vi "Mix Columns-PORTABLE-5129.vi"(7 "State In":u16[][](array[numeric])=[[45, 83, 174, 45], [73, 86, 101, 162], [176, 106, 51, 68], [108, 81, 250, 240]], 11 "error in":errorcluster) -> (8 "State Out":u16[][](array[numeric]), 15 "error out":errorcluster)   [LabVIEW 2020, in "Library Commun.lvlib"]
doc: "In the MixColumns step, the four bytes of each column of the state are combined using an invertible linear transformation. The MixColumns step can also be viewed as a multiplication by a particular MDS matrix in a finite field.\n\n<inline>"
uses:
  Library Commun.lvlib
panel:
  in  "0x011b":u16=283 format="%.0x"
  in  "0x80":u16=128 format="%.0x"
  # "old s= 45,83,174,45,73,86,101,162,176,106,51,68,108,81,250,240"
  # "new s= 93,103,33,19,24,16,203,78,171,34,184,12,86,107,80,106"
  # "255,97,23,96,160,73,200,160,172,154,205,24,        180,50,93,135"
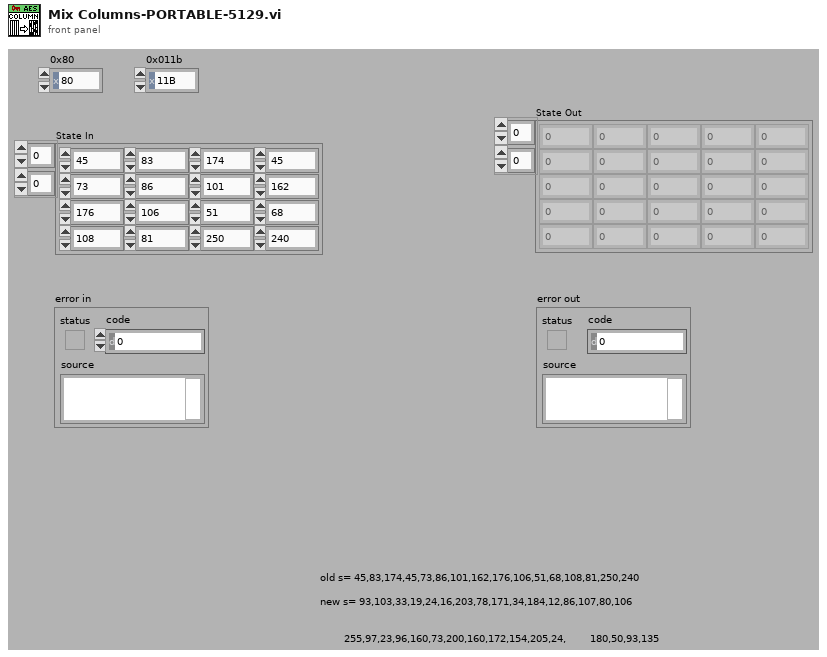
[diagram p1: front panel]
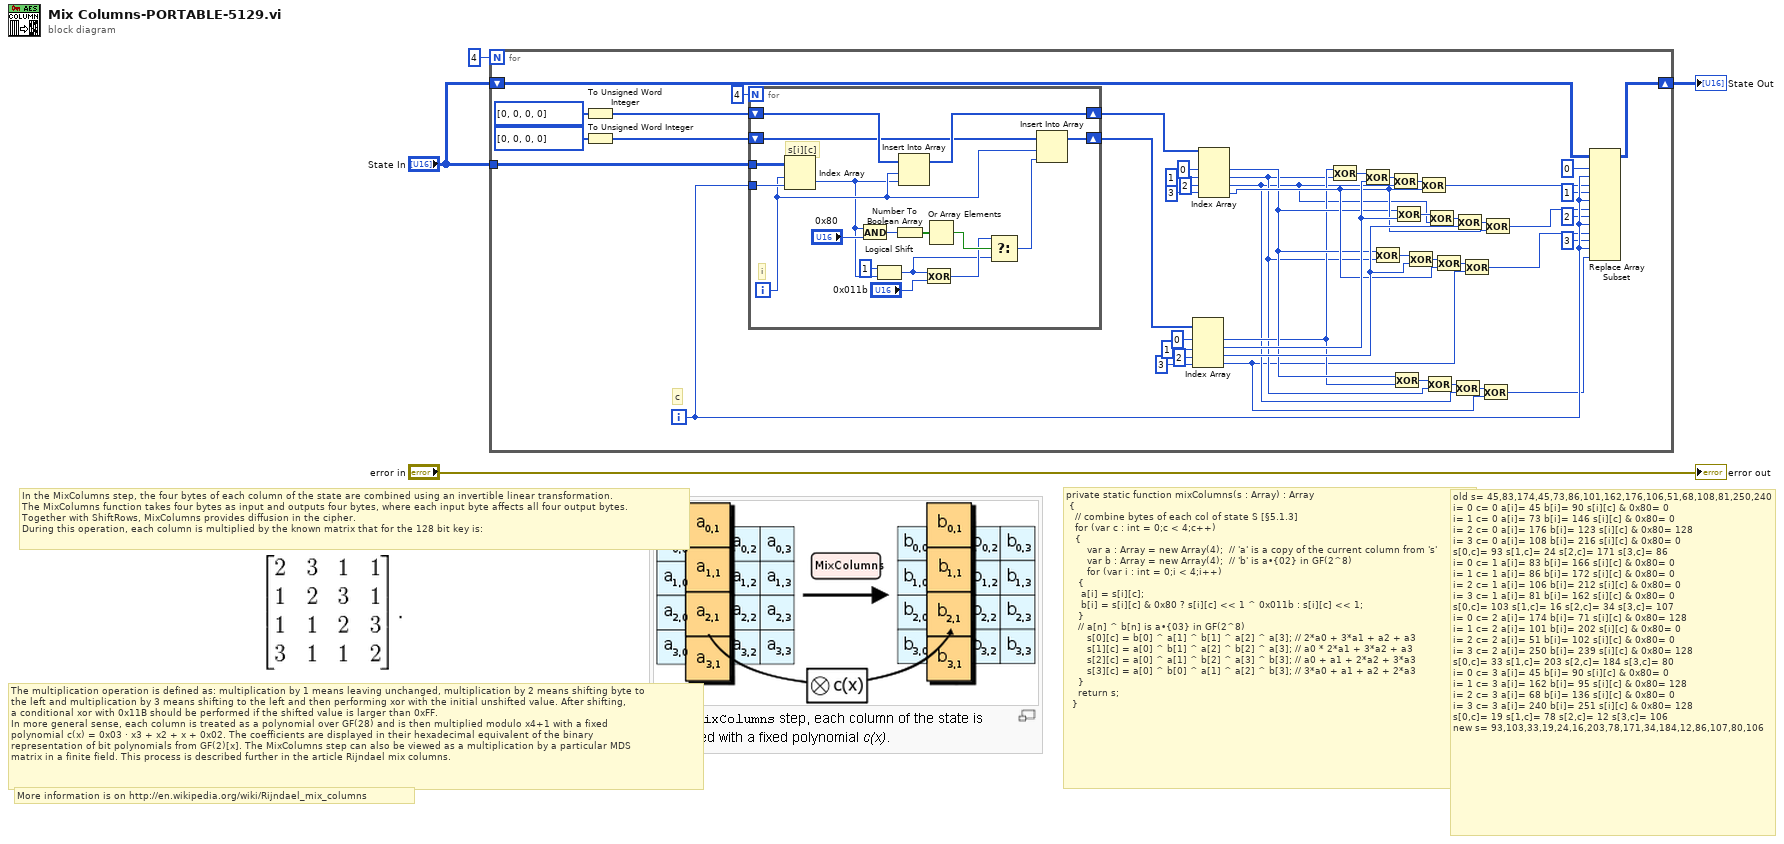
[diagram p0: block diagram]
diagram:
  # "More information is on http://en.wikipedia.org/wiki/Rijndael_mix_columns"
  # "The multiplication operation is defined as: multiplication by 1 means leaving unchanged, multiplication by 2 means shifting byte to\nthe left and multiplication by 3 means shifting to the left and then performing xor with the initial unshifted value. After shifting, \na conditional xor with 0x11B should be performed if the shifted value is larger than 0xFF.\nIn more general sense, each column is treated as a polynomial over GF(28) and is then multiplied modulo x4+1 with a fixed \npolynomial c(x) = 0x03 · x3 + x2 + x + 0x02. The coefficients are displayed in their hexadecimal equivalent of the binary \nrepresentation of bit polynomials from GF(2)[x]. The MixColumns step can also be viewed as a multiplication by a particular MDS \nmatrix in a finite field. This process is described further in the article Rijndael mix columns."
  # "In the MixColumns step, the four bytes of each column of the state are combined using an invertible linear transformation.\nThe MixColumns function takes four bytes as input and outputs four bytes, where each input byte affects all four output bytes.\nTogether with ShiftRows, MixColumns provides diffusion in the cipher.\nDuring this operation, each column is multiplied by the known matrix that for the 128 bit key is:"
  # "old s= 45,83,174,45,73,86,101,162,176,106,51,68,108,81,250,240\ni= 0 c= 0 a[i]= 45 b[i]= 90 s[i][c] & 0x80= 0\ni= 1 c= 0 a[i]= 73 b[i]= 146 s[i][c] & 0x80= 0\ni= 2 c= 0 a[i]= 176 b[i]= 123 s[i][c] & 0x80= 128\ni= 3 c= 0 a[i]= 108 b[i]= 216 s[i][c] & 0x80= 0\ns[0,c]= 93 s[1,c]= 24 s[2,c]= 171 s[3,c]= 86\ni= 0 c= 1 a[i]= 83 b[i]= 166 s[i][c] & 0x80= 0\ni= 1 c= 1 a[i]= 86 b[i]= 172 s[i][c] & 0x80= 0\ni= 2 c= 1 a[i]= 106 b[i]= 212 s[i][c] & 0x80= 0\ni= 3 c= 1 a[i]= 81 b[i]= 162 s[i][c] & 0x80= 0\ns[0,c]= 103 s[1,c]= 16 s[2,c]= 34 s[3,c]= 107\ni= 0 c= 2 a[i]= 174 b[i]= 71 s[i][c] & 0x80= 128\ni= 1 c= 2 a[i]= 101 b[i]= 202 s[i][c] & 0x80= 0\ni= 2 c= 2 a[i]= 51 b[i]= 102 s[i][c] & 0x80= 0\ni= 3 c= 2 a[i]= 250 b[i]= 239 s[i][c] & 0x80= 128\ns[0,c]= 33 s[1,c]= 203 s[2,c]= 184 s[3,c]= 80\ni= 0 c= 3 a[i]= 45 b[i]= 90 s[i][c] & 0x80= 0\ni= 1 c= 3 a[i]= 162 b[i]= 95 s[i][c] & 0x80= 128\ni= 2 c= 3 a[i]= 68 b[i]= 136 s[i][c] & 0x80= 0\ni= 3 c= 3 a[i]= 240 b[i]= 251 s[i][c] & 0x80= 128\ns[0,c]= 19 s[1,c]= 78 s[2,c]= 12 s[3,c]= 106\nnew s= 93,103,33,19,24,16,203,78,171,34,184,12,86,107,80,106"
  # "private static function mixColumns(s : Array) : Array \n {   \n\t\t\t// combine bytes of each col of state S [§5.1.3]\n\t\t\tfor (var c : int = 0;c < 4;c++) \n\t\t\t{\n\t\t\t\t   var a : Array = new Array(4);  // 'a' is a copy of the current column from 's'\n\t\t\t\t   var b : Array = new Array(4);  // 'b' is a•{02} in GF(2^8)\n\t\t\t   \tfor (var i : int = 0;i < 4;i++) \n\t\t\t\t{\n\t\t\t\t\ta[i] = s[i][c];\n\t\t\t\t\tb[i] = s[i][c] & 0x80 ? s[i][c] << 1 ^ 0x011b : s[i][c] << 1;\n\t\t\t\t}\n\t\t\t\t// a[n] ^ b[n] is a•{03} in GF(2^8)\n\t\t\t\t   s[0][c] = b[0] ^ a[1] ^ b[1] ^ a[2] ^ a[3]; // 2*a0 + 3*a1 + a2 + a3\n\t\t\t\t   s[1][c] = a[0] ^ b[1] ^ a[2] ^ b[2] ^ a[3]; // a0 * 2*a1 + 3*a2 + a3\n\t\t\t   \ts[2][c] = a[0] ^ a[1] ^ b[2] ^ a[3] ^ b[3]; // a0 + a1 + 2*a2 + 3*a3\n\t\t\t   \ts[3][c] = a[0] ^ b[0] ^ a[1] ^ a[2] ^ b[3]; // 3*a0 + a1 + a2 + 2*a3\n\t\t\t\t}\n\t\t\t\treturn s;\n\t\t}"
  n1 = for {
    N: 4 -> [_]
    shift-right: [w48] -> w2
    shift-left: "State In" -> [w49]
    tunnel: "State In" -> [w50]
    i -> [w51]
    # "c"
    n2 = To Unsigned Word Integer(number=i32[] [0, 0, 0, 0] ("t[c]")) -> (unsigned 16bit integer=w45:u16[])
    n3 = To Unsigned Word Integer(number=i32[] [0, 0, 0, 0] ("t[c]")) -> (unsigned 16bit integer=w44:u16[])
    n4 = for {
      N: 4 -> [_]
      tunnel: w50 -> [w68]
      tunnel: w51 -> [w67]
      shift-right: [w54] -> w43
      shift-left: w45 -> [w55]
      shift-right: [w52] -> w42
      shift-left: w44 -> [w53]
      i -> [w66]
      # "s[i][c]"
      # "i"
      n5 = Index Array(array=w68, index (row)=w66, index (col)=w67) -> (element=w60:u16)
      n6 = And(x=w60, y="0x80") -> (x .and. y?=w63:u16)
      n7 = Logical Shift(y=i8 1, x=w60) -> (x << y=w57:u16)
      n8 = Number To Boolean Array(number=w63) -> (Boolean array=w62:bool[])
      n9 = Insert Into Array(array=w55, index=w66, new element=w60) -> (w54:u16[])
      n10 = Exclusive Or(1:"0x011b", 2:w57) -> (0:w58:u16)
      n11 = Or Array Elements(Boolean array=w62) -> (logical OR=w61:bool)
      n12 = Select(t=w58, s=w61, f=w57) -> (s? t:f=w65:u16)
      n13 = Insert Into Array(array=w53, index=w66, new element=w65) -> (w52:u16[])
    }
    n14 = Index Array(array=w42, index #1=0 ("index"), index #2=1 ("index"), index #3=2 ("index"), index #4=3 ("index")) -> (element #1=w13:u16, element #2=w25:u16, element #3=w20:u16, element #4=w10:u16)
    n15 = Index Array(array=w43, index #1=0 ("index"), index #2=1 ("index"), index #3=2 ("index"), index #4=3 ("index")) -> (element #1=w14:u16, element #2=w12:u16, element #3=w11:u16, element #4=w19:u16)
    n16 = Exclusive Or(1:w12, 2:w13) -> (0:w32:u16)
    n17 = Exclusive Or(1:w25, 2:w32) -> (0:w31:u16)
    n18 = Exclusive Or(1:w12, 2:w14) -> (0:w23:u16)
    n19 = Exclusive Or(1:w11, 2:w31) -> (0:w30:u16)
    n20 = Exclusive Or(1:w13, 2:w14) -> (0:w17:u16)
    n21 = Exclusive Or(1:w25, 2:w14) -> (0:w28:u16)
    n22 = Exclusive Or(1:w20, 2:w23) -> (0:w22:u16)
    n23 = Exclusive Or(1:w19, 2:w30) -> (0:w29:u16)
    n24 = Exclusive Or(1:w12, 2:w17) -> (0:w16:u16)
    n25 = Exclusive Or(1:w11, 2:w28) -> (0:w27:u16)
    n26 = Exclusive Or(1:w19, 2:w22) -> (0:w21:u16)
    n27 = Exclusive Or(1:w11, 2:w16) -> (0:w15:u16)
    n28 = Exclusive Or(1:w20, 2:w27) -> (0:w26:u16)
    n29 = Exclusive Or(1:w10, 2:w21) -> (0:w18:u16)
    n30 = Exclusive Or(1:w10, 2:w15) -> (0:w9:u16)
    n31 = Exclusive Or(1:w19, 2:w26) -> (0:w24:u16)
    n32 = Replace Array Subset(array=w49, new element #1=w29, index (row) #1=0 ("disabled index (col)"), index (col) #1=w51, new element #2=w24, index (row) #2=1 ("disabled index (col)"), index (col) #2=w51, new element #3=w18, index (row) #3=2 ("disabled index (col)"), index (col) #3=w51, new element #4=w9, index (row) #4=3 ("disabled index (col)"), index (col) #4=w51) -> (w48:u16[][])
  }
  "State Out" <- w2
  "error out" <- "error in"
